vi "Switch Mode STM-AFM.vi"() -> ()   [LabVIEW 2016]
doc: "This example switches between STM and AFM modes.\n \n\n- Nanonis Programming Interface -"
uses:
  Nanonis Prog Interface.lvlib
panel:
  in  "Tip Lift (m)":sgl=5e-08 format="%_5p"
  in  "Excitation Output":bool=TRUE
  in  "AFM Bias":sgl format="%_5p"
  in  "STM Bias":sgl=1.0 format="%_5p"
  in  "Phase Controller":bool
  in  "Amplitude Controller":bool=TRUE
  in  "AFM Controller name":string="Frequency (neg)"
  in  "STM Controller name":string="log Current"
  in  "Switch to":bool=TRUE
  # "STM"
  # "AFM"
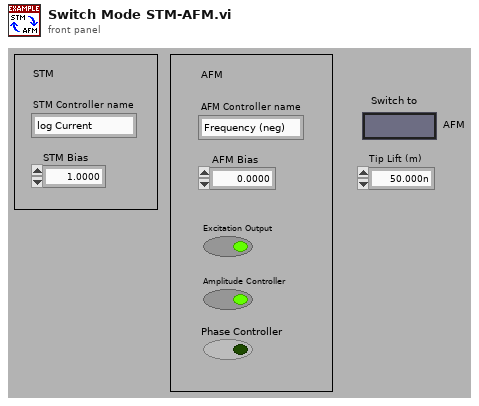
[diagram p1: front panel]
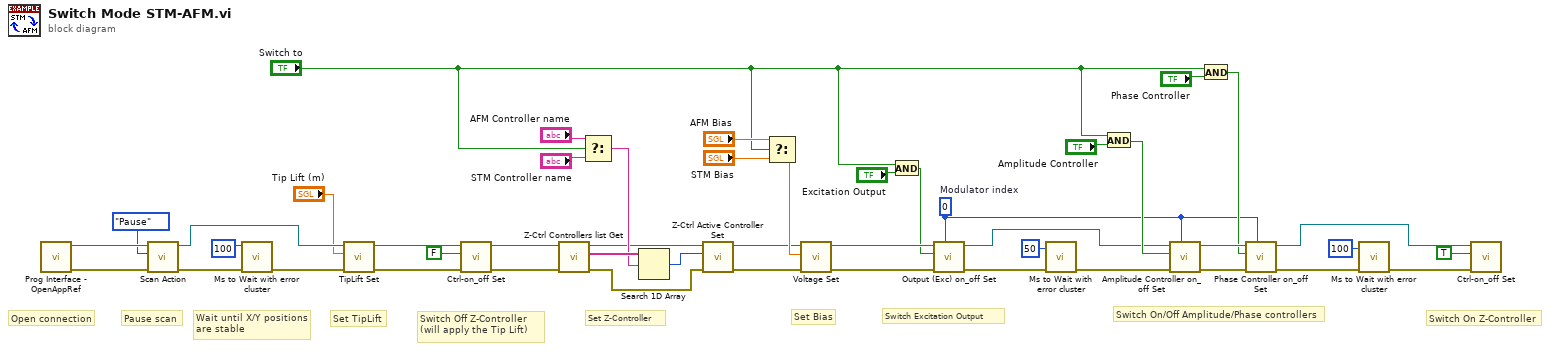
[diagram p0: block diagram]
diagram:
  w1 = 0  # Modulator index
  # "Set TipLift"
  # "Switch On Z-Controller"
  # "Switch On/Off Amplitude/Phase controllers"
  # "Switch Excitation Output"
  # "Set Z-Controller"
  # "Set Bias"
  # "Wait until X/Y positions \nare stable"
  # "Switch Off Z-Controller\n(will apply the Tip Lift)"
  # "Pause scan"
  # "Open connection"
  n1 = call <userlib>:"Prog Interface - OpenAppRef.vi"() -> ("Error out"=w45:errorcluster, "Application reference"=w46:refnum<vi>)  [unwired: 6 in]
  n2 = call <userlib>:"Scan Action.vi"("error in (no error)"=w45, "Scan action (Start)"=enum16{"Start", "Stop", "Pause", "Resume"}."Pause", "Application ref in"=w46) -> ("error out"=w40:errorcluster, "Application ref out"=w24:refnum<vi>)  [unwired: 6 in]
  n3 = call "Ms to Wait with error cluster.vi"("error in (no error)"=w40, "milliseconds to wait"=u32 100 ("ms to wait after stop scan")) -> ("error out"=w23:errorcluster)  [unwired: 4 in, 1 out]
  n4 = call <userlib>:"TipLift Set.vi"("error in (no error)"=w23, "TipLift (m)"="Tip Lift (m)", "Application ref in"=w24) -> ("error out"=w22:errorcluster, "Application ref out"=w21:refnum<vi>)  [unwired: 7 in]
  n5 = call <userlib>:"Ctrl-on_off Set.vi"("error in (no error)"=w22, "Z Controller ON/OFF"=FALSE, "Application ref in"=w21) -> ("error out"=w18:errorcluster, "Application ref out"=w17:refnum<vi>)  [unwired: 7 in]
  n6 = call <userlib>:"Z-Ctrl Controllers list Get.vi"("error in (no error)"=w18, "Application ref in"=w17) -> ("error out"=w37:errorcluster, "Z Controllers list"=w43:string[], "Application ref out"=w36:refnum<vi>)  [unwired: 6 in, 1 out]
  n7 = Select(t="AFM Controller name", s="Switch to", f="STM Controller name") -> (s? t:f=w38:string)
  n8 = Search 1D Array(1D array=w43, element=w38) -> (index of element=w39:i32)  [unwired: 1 in]
  n9 = call <userlib>:"Z-Ctrl Active Controller Set.vi"("error in (no error)"=w37, "Z Controller index"=w39, "Application ref in"=w36) -> ("error out"=w15:errorcluster, "Application ref out"=w16:refnum<vi>)  [unwired: 7 in]
  n10 = Select(t="AFM Bias", s="Switch to", f="STM Bias") -> (s? t:f=w19:sgl)
  n11 = call <userlib>:"Voltage Set.vi"("Error in (no error)"=w15, "Bias (V)"=w19, "Application ref in"=w16) -> ("Error out"=w14:errorcluster, "Application ref out"=w13:refnum<vi>)  [unwired: 7 in]
  n12 = And(x="Switch to", y="Excitation Output") -> (x .and. y?=w12:bool)
  n13 = call <userlib>:"Output (Exc) on_off Set.vi"("Modulator index"=w1, "Error in (no error)"=w14, "Output ON/OFF (F=OFF)"=w12, "Application ref in"=w13) -> ("Error out"=w9:errorcluster, "Application ref out"=w7:refnum<vi>)  [unwired: 6 in]
  n14 = call "Ms to Wait with error cluster.vi"("error in (no error)"=w9, "milliseconds to wait"=u32 50 ("ms to wait after stop scan")) -> ("error out"=w8:errorcluster)  [unwired: 4 in, 1 out]
  n15 = And(x="Switch to", y="Amplitude Controller") -> (x .and. y?=w28:bool)
  n16 = call <userlib>:"Amplitude Controller on_off Set.vi"("Modulator index"=w1, "Error in (no error)"=w8, "Amplitude controller ON/OFF"=w28, "Application ref in"=w7) -> ("Error out"=w34:errorcluster, "Application ref out"=w35:refnum<vi>)  [unwired: 6 in]
  n17 = And(x="Switch to", y="Phase Controller") -> (x .and. y?=w27:bool)
  n18 = call <userlib>:"Phase Controller on_off Set.vi"("Modulator index"=w1, "Error in (no error)"=w34, "Phase controller ON/OFF"=w27, "Application ref in"=w35) -> ("Error out"=w3:errorcluster, "Application ref out"=w4:refnum<vi>)  [unwired: 6 in]
  n19 = call "Ms to Wait with error cluster.vi"("error in (no error)"=w3, "milliseconds to wait"=u32 100 ("ms to wait after stop scan")) -> ("error out"=w2:errorcluster)  [unwired: 4 in, 1 out]
  n20 = call <userlib>:"Ctrl-on_off Set.vi"("error in (no error)"=w2, "Z Controller ON/OFF"=TRUE, "Application ref in"=w4) -> ()  [unwired: 7 in, 2 out]
